vi "RemovePackageFromCEPMFeed.vi"(8 "Error In":errorcluster, 11 "Package Path":path) -> (0 "Error Out":errorcluster)   [LabVIEW 2019, in "CEPM.lvlib"]
uses:
  CEPM.lvlib
  <vilib>/National Instruments/NIPM API (Beta)/NIPM_API.lvlib
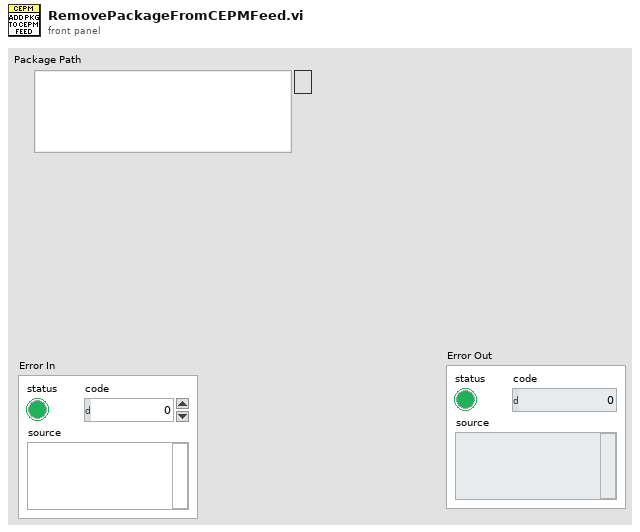
[diagram p1: front panel]
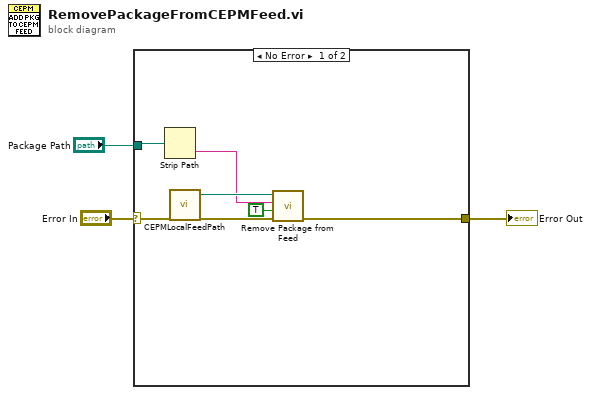
[diagram p0: block diagram]
diagram:
  n1 = case shown="No Error" "Error In" {
    selector: "Error In" -> [w10 w11]
    tunnel: [w7 w11] -> w2
    tunnel: "Package Path" -> [w6 _]
    frame No Error {
      n2 = Strip Path(path=w6) -> (name=w5:string)  [unwired: 1 out]
      n3 = call "CEPMLocalFeedPath.vi"("Error In"=w10) -> ("Error Out"=w8:errorcluster, "CEPM Local Feed Path"=w9:path)  [unwired: 9 in]
      n4 = call <vilib>:"Remove Package from Feed.vi"("error in"=w8, "delete package file? (F)"=TRUE, "package filename"=w5, "feed folderpath in"=w9) -> ("error out"=w7:errorcluster)  [unwired: 4 in, 3 out]
    }
    frame Error {
    }
  }
  "Error Out" <- w2
